vi "初始化数组.vi"() -> ()   [LabVIEW 2012]
panel:
  out "空数组":dbl[](array[numeric])
  out "初始化的数组 2":bool[][](array[boolean])
  out "初始化的数组":dbl[](array[numeric])
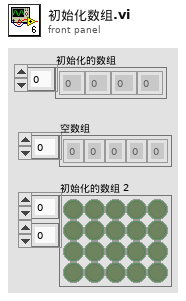
[diagram p1: front panel]
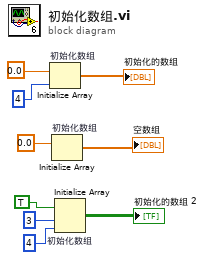
[diagram p0: block diagram]
diagram:
  n1 = Initialize Array "初始化数组"(0.0 ("元素"), 4 ("维数大小")) -> (→"初始化的数组":dbl[])
  n2 = Initialize Array "初始化数组"(0.0 ("元素")) -> (→"空数组":dbl[])  [unwired: 1 in]
  n3 = Initialize Array "初始化数组"(TRUE, 3 ("维数大小"), 4 ("维数大小")) -> (→"初始化的数组 2":bool[][])
